vi "FINS In-read.vi"(0 "FINS Header i":T1 {"SNA" max=127 format="%x"; "SA2" max=254 step=1 format="%x"; "SA1" format="%x"; "DA2" max=254 step=1 format="%x"; "DA1" format="%x"; "DNA" max=127 step=1 format="%x"}, 5 "msg 3":string, 11 "error i":errorcluster) -> (4 "FINS Header o":T1 {"SNA" max=127 format="%x"; "SA2" max=254 step=1 format="%x"; "SA1" format="%x"; "DA2" max=254 step=1 format="%x"; "DA1" format="%x"; "DNA" max=127 step=1 format="%x"}, 8 "data":u8[](array[numeric]), 10 "data":bool[][](array[boolean]), 12 "CMD":T2, 13 "FINS Header 2":T1={"resp req"=FALSE, "cmd resp"=FALSE, "SID"=255, "DNA"=2, "DA1"=2, "DA2"=2, "SA1"=0, "SA2"=255, "SNA"=255} {"SNA" max=127 format="%x"; "SA2" max=254 step=1 format="%x"; "SA1" format="%x"; "DA2" max=254 step=1 format="%x"; "DA1" format="%x"; "DNA" max=127 step=1 format="%x"}, 14 "RSP":bool, 15 "error o":errorcluster)   [LabVIEW 2019]
uses:
  FINS/FINS_header.ctl
  FINS/FINS CMD.ctl
  FINS/FINS TCP.lvlib
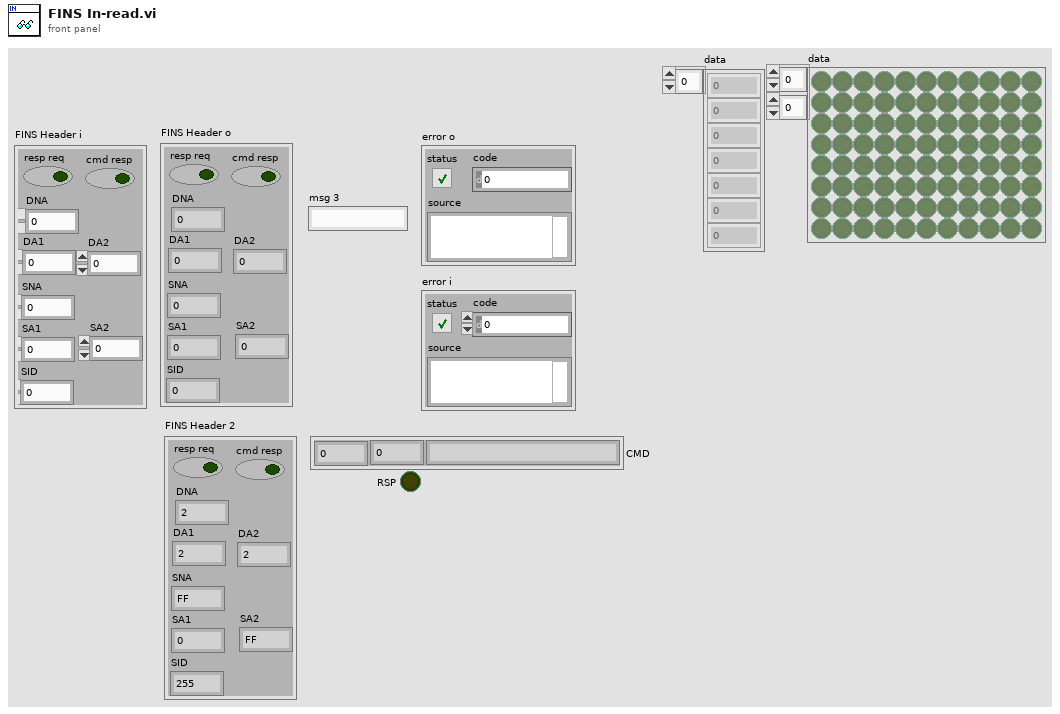
[diagram p1: front panel]
types:
  T1 = typedef "FINS TCP.lvlib/FINS_header.ctl" = cluster{"resp req":bool, "cmd resp":bool, "SID":u8, "DNA":u8, "DA1":u8, "DA2":u8, "SA1":u8, "SA2":u8, "SNA":u8}
  T2 = typedef "FINS TCP.lvlib/FINS CMD.ctl" = cluster{"MR":u8, "SR":u8, "name":string}
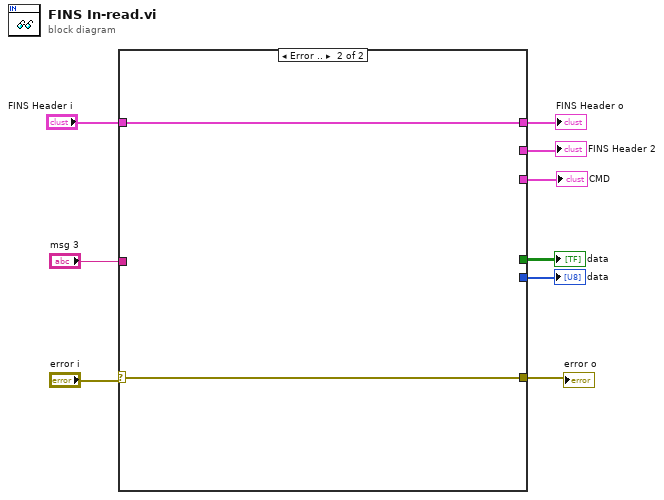
[diagram p0: block diagram]
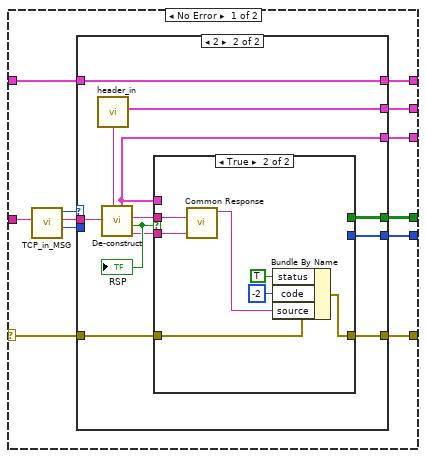
[diagram p2: hidden frame]
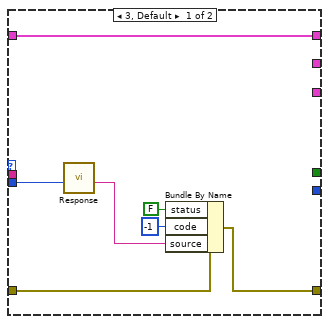
[diagram p3: hidden frame]
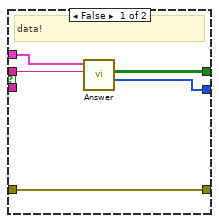
[diagram p4: hidden frame]
diagram:
  n1 = case shown="Error .." "error i" {
    selector: "error i" -> [w16 w54]
    tunnel: "msg 3" -> [w21 _]
    tunnel: [w15 w54] -> w7
    tunnel: "FINS Header i" -> [w19 w53]
    tunnel: [w20 w53] -> w5
    tunnel: [w13 _] -> w4
    tunnel: [w12 _] -> w3
    tunnel: [w11 _] -> w2
    tunnel: [w10 _] -> w1
    frame No Error {
      n2 = call "TCP_in_MSG.vi"("msg i"=w21) -> ("rsp"=w17:u32, "msg o"=w14:string, "cmd"=w18:u32)  [unwired: 8 in]
      n3 = case shown="2" w18 {
        tunnel: [w26 w40] -> w20
        tunnel: w19 -> [w26 w40]
        tunnel: w17 -> [w28 _]
        tunnel: w16 -> [w27 w32]
        tunnel: [w25 w31] -> w15
        tunnel: w14 -> [_ w35]
        tunnel: [_ w34] -> w13
        tunnel: [_ w33] -> w12
        tunnel: [_ w30] -> w11
        tunnel: [_ w29] -> w10
        frame 3, Default {
          n4 = call "Response.vi"("rsp"=w28) -> ("error"=w22:string)  [unwired: 10 in]
          n5 = Bundle By Name(cluster=w27, "status"=FALSE, "code"=-1, "source"=w22) -> (w25:errorcluster)
        }
        frame 2 {
          n6 = call "De-construct.vi"("msg o"=w35) -> ("MSES/SRES"=w36:string, "RSP?"=w39:bool, "Data"=w38:string, "CMD"=w34:T2, "header"=w37:string)  [unwired: 6 in]
          "RSP" <- w39
          n7 = call "header_in.vi"("HEADER"=w37) -> ("FINS Header"=w33:T1)  [unwired: 10 in]
          n8 = case shown="True" w39 {
            tunnel: w36 -> [_ w51]
            tunnel: w38 -> [w44 w52]
            tunnel: w34 -> [w45 _]
            tunnel: w32 -> [w43 w48]
            tunnel: [w43 w47] -> w31
            tunnel: [w42 _] -> w30
            tunnel: [w41 _] -> w29
            frame False {
              # "data!"
              n9 = call "Answer.vi"("Data"=w44, "CMD 2"=w45) -> ("dec"=w41:u8[], "Boolean array"=w42:bool[][])  [unwired: 8 in]
            }
            frame True {
              n10 = call "Common Response.vi"("RSP"=w51, "Data"=w52) -> ("error"=w46:string)  [unwired: 6 in, 3 out]
              n11 = Bundle By Name(cluster=w48, "status"=TRUE, "code"=-2, "source"=w46) -> (w47:errorcluster)
            }
          }
        }
      }
    }
    frame Error {
    }
  }
  "FINS Header o" <- w5
  "error o" <- w7
  "FINS Header 2" <- w3
  "CMD" <- w4
  "data" <- w2
  "data" <- w1
